vi "Tx5xx-Ethernet.vi"() -> ()   [LabVIEW 2013]
doc: "Use this template to create an application that executes repeatedly until you click the Stop button. This template polls the state of the Stop button and does not use events. Use the Top-Level Application template (not available in the Base package) to create a single-loop application with event handling."
uses:
  NI Modbus.llb/MB Modbus Command.ctl
  Instance           1 33Saved   SingleLoopApplication.vit .vi
panel:
  out "Registers":u16[](array[numeric]) format="%04x"
  in  "Tab Control":enum32{"Setup", "Graphs"}(tab)
  out "Relative humidity":dbl(knob) scale=0.0..100.0
  in  "stop":bool
  in  "Delay Time (s)":dbl=1.0
  out "Measured values":T1 {"Temperature" format="%.1f"; "Relative humidity" format="%.1f"; "Computed value" format="%.1f"; "Pressure" format="%.1f"}
  out "Temperature":dbl(slide) scale=10.0..35.0 scale format="%#.1p"
  out "Pressure 2":dbl(knob) caption="Barometric pressure" scale=900.0..1100.0
  in  "Remote Port":u16=502
  in  "Remote IP Address":string="192.168.1.213"
  in  "Modbus Command":T2={"Function Code"=3, "Starting Address"=48, "Quantity"=4, "Data"=[], "Discrete"=[]} {"Function Code" items=["Read Coils"=1, "Read Discrete Inputs"=2, "Read Holding Registers"=3, "Read Input Registers"=4, "Write Single Coil"=5, "Write Single Register"=6, "Read Exception Status"=7, "Write Multiple Coils"=15, "Write Multiple Registers"=16]}
  out "connection ID":refnum<k5>
  out "Relative humidity":dbl(graph)
  out "Temperature":dbl(graph)
  out "Computed Value":dbl(graph)
  out "Pressure":dbl(graph)
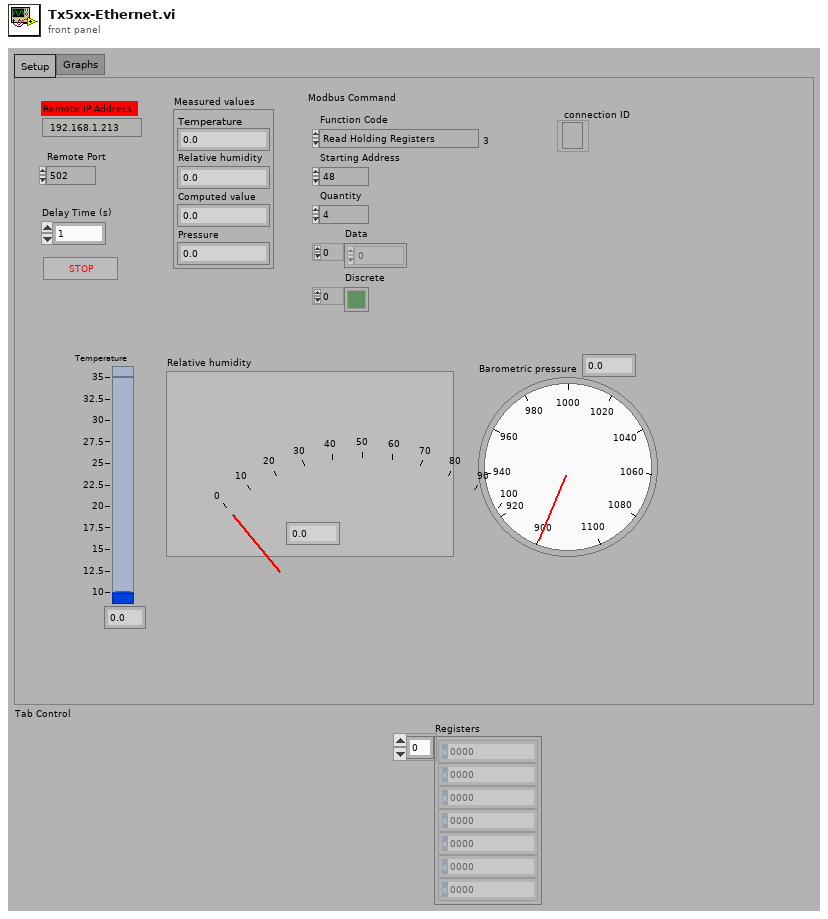
[diagram p1: front panel]
types:
  T1 = cluster{"Temperature":dbl, "Relative humidity":dbl, "Computed value":dbl, "Pressure":dbl}
  T2 = typedef "MB Modbus Command.ctl" = cluster{"Function Code":u8, "Starting Address":u16, "Quantity":u16, "Data":u16[], "Discrete":bool[]}
  T3 = cluster{"[0]":dbl, "[1]":dbl, "[2]":dbl, "[3]":dbl}
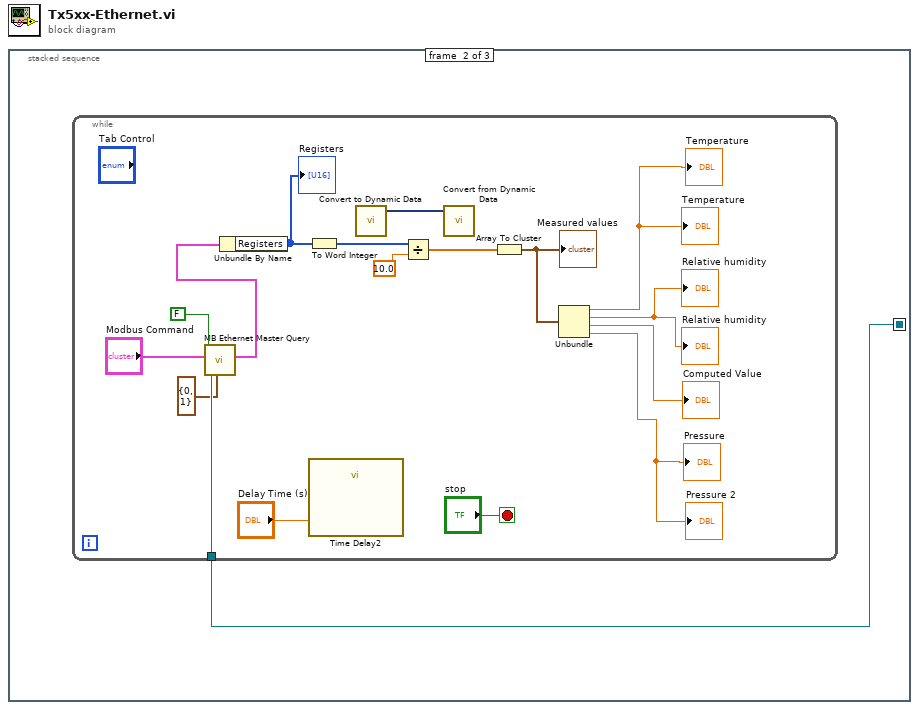
[diagram p0: block diagram]
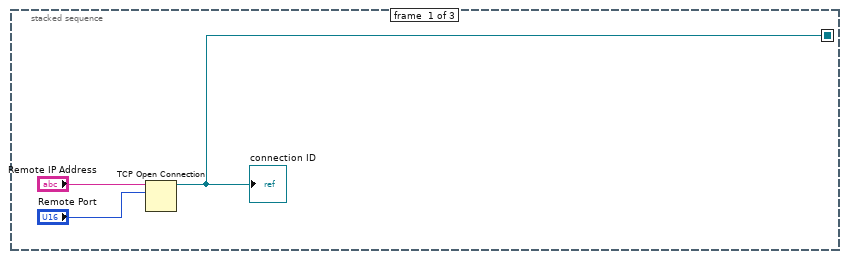
[diagram p2: hidden frame]
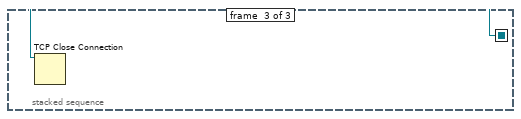
[diagram p3: hidden frame]
diagram:
  n1 = stacked-sequence {
    seq-local: [w1 _ _] -> [_ w4 w22]
    frame #0 {
      n2 = TCP Open Connection(address="Remote IP Address", remote port or service name="Remote Port") -> (connection ID=w1:refnum<k5>)  [unwired: 3 in, 1 out]
      "connection ID" <- w1
    }
    frame #1 {
      n3 = while {
        tunnel: w4 -> [w9]
        stop <- "stop" stop-if-true
        n4 = call "MB Ethernet Master Query.vi"("MBAP Header"=cluster{"Transaction ID":u16, "Unit ID":u8} {"Transaction ID"=0, "Unit ID"=1}, "Use MODBUS Data Unit?"=FALSE, "Modbus Command"="Modbus Command", "TCP Connection Refnum in"=w9) -> ("Registers"=w10:cluster{"Registers":u16[], "Discrete":bool[]})  [unwired: 3 in, 4 out]
        n5 = Unbundle By Name(w10) -> ("Registers"=w18:u16[])
        "Registers" <- w18
        n6 = To Word Integer(number=w18) -> (16bit integer=w6:i16[])
        n7 = call "Time Delay2"("Delay Time (s)"="Delay Time (s)") -> ()  [unwired: 10 in, 1 out]
        n8 = call "Convert to Dynamic Data"() -> ("Dynamic Data Type"=w7:dynamicdata)  [unwired: 4 in]
        n9 = Divide(x=w6, y=10.0) -> (x/y=w5:dbl[])
        n10 = call "Convert from Dynamic Data"("Dynamic Data Type"=w7) -> ()  [unwired: 3 in, 1 out]
        n11 = Array To Cluster(array=w5) -> (cluster=w17:T3)
        "Measured values" <- w17
        n12 = Unbundle(w17) -> ("[0]"=→"Temperature" →"Temperature":dbl, "[1]"=→"Relative humidity" →"Relative humidity":dbl, "[2]"=→"Computed Value":dbl, "[3]"=→"Pressure" →"Pressure 2":dbl)
      }
    }
    frame #2 {
      n13 = TCP Close Connection(connection ID=w22) -> ()  [unwired: 2 in, 2 out]
    }
  }
